vi "Actor Core.vi"(8 "error in":errorcluster, 11 "Sounds in":refnum<class "Sounds.lvclass">) -> (0 "error out":errorcluster, 3 "Actor out":refnum<class "Actor.lvclass">)   [LabVIEW 2021, in "Sounds.lvlib" / "Sounds.lvclass"]
doc: "<p>(<strong>Filename</strong>: <span class=\"dnl\">Actor Framework.lvlib:Actor.lvclass:Actor Core.vi</span>)</p>\n<p>Receives messages to the actor, reacts to them, and initiates any error handling that may shut the actor down.</p>\n<p>Descendant classes may override this VI to append parallel tasks for the actor to complete while it handles messages. Overrides use the <a href=\"nihelplauncher://docs/csh?context=lvcore_glang_udclass\">Call Parent Class Method</a> node.</p>"
uses:
  Sounds.lvclass
  C:/Program Files/National Instruments/LabVIEW 2024/vi.lib/ActorFramework/Actor/Actor.lvclass
  <vilib>/ActorFramework/Actor/Actor.lvclass
  <vilib>/ActorFramework/Actor/Actor.lvclass/Actor.ctl
  <vilib>/ActorFramework/Message Enqueuer/Message Enqueuer.lvclass/Message Enqueuer.ctl
  <vilib>/ActorFramework/Message Enqueuer/Init from Existing Queue.vi
  <vilib>/ActorFramework/Message Enqueuer/Enqueue.vi
  Sounds Messages/Start Playing Msg/Start Playing Msg.lvclass
  C:/Program Files/National Instruments/LabVIEW 2024/vi.lib/ActorFramework/Message/Message.lvclass
  <vilib>/ActorFramework/Message Priority Queue/Priority Enqueue.vi
  <vilib>/ActorFramework/Message Enqueuer/Message Enqueuer.lvclass
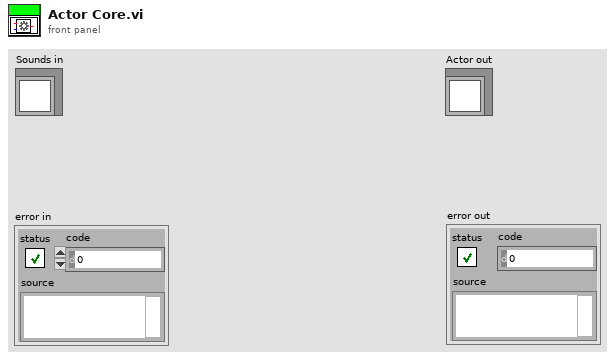
[diagram p1: front panel]
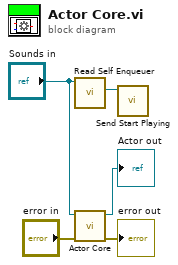
[diagram p0: block diagram]
diagram:
  n1 = call <vilib>:"Read Self Enqueuer.vi"("Actor"="Sounds in") -> ("Self Enqueuer"=w1:refnum<class "Message Enqueuer.lvclass">)  [unwired: 10 in]
  n2 = call-parent "Actor Core.vi"("error in"="error in", "Actor in"="Sounds in") -> ("error out"=→"error out":errorcluster, "Actor out"=→"Actor out":refnum<class "Actor.lvclass">)  [unwired: 8 in]
  n3 = call "Send Start Playing.vi"("Message Enqueuer"=w1) -> ()  [unwired: 9 in, 2 out]
